vi "Close Write Reference.vi"(8 "error in":errorcluster, 11 "TDMS in":refnum<class "TDMS.lvclass">) -> (0 "error out":errorcluster, 3 "TDMS out":refnum<class "TDMS.lvclass">)   [LabVIEW 2019, in "TDMS.lvlib" / "TDMS.lvclass"]
uses:
  TDMS.lvclass
  C:/Users/Public/Documents/Development/builds/Tools/Report.lvlibp/Report.lvclass
  TDMS.lvclass/TDMS.ctl
  Accessors/Read TDMS Ref.vi
  builds/Tools/Report.lvlibp/Accessors/Write Root Path.vi
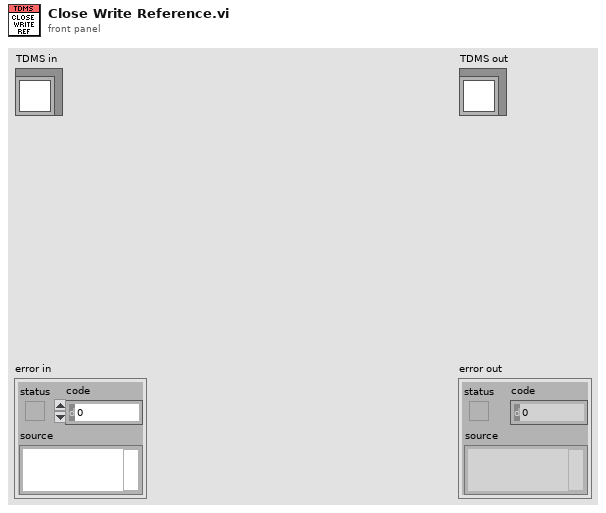
[diagram p1: front panel]
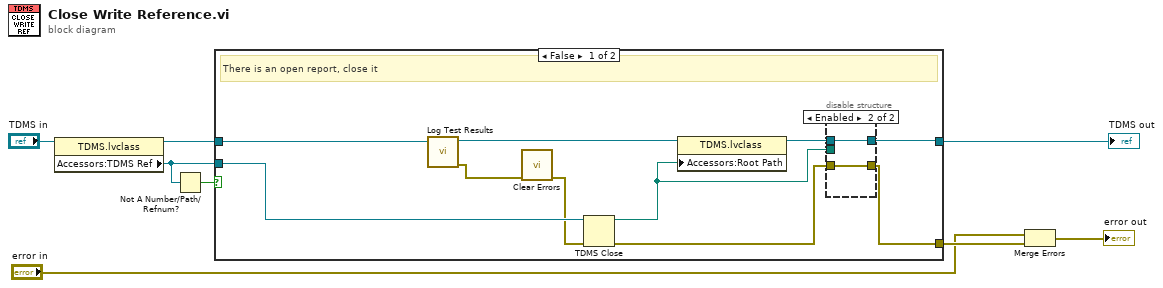
[diagram p0: block diagram]
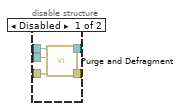
[diagram p2: hidden frame]
diagram:
  n1 = property class="TDMS.lvclass"(reference="TDMS in") -> (reference out=w5:refnum<class "TDMS.lvclass">, "Accessors:TDMS Ref"=w4:refnum<k34>)  [unwired: 1 in, 1 out]
  n2 = Not A Number/Path/Refnum?(number/path/refnum=w4) -> (NaN/Path/Refnum?=w6:bool)
  n3 = case shown="False" w6 {
    tunnel: w5 -> [w18 w26]
    tunnel: w4 -> [w17 _]
    tunnel: [w12 w26] -> w3
    tunnel: [w10 _] -> w2
    frame False {
      # "There is an open report, close it"
      n4 = call "Log Test Results.vi"("TDMS in"=w18) -> ("error out"=w14:errorcluster, "TDMS out"=w15:refnum<class "TDMS.lvclass">)  [unwired: 9 in]
      n5 = call <vilib>:"Clear Errors.vi"("error in (no error)"=w14) -> ("error out"=w16:errorcluster)  [unwired: 5 in, 1 out]
      n6 = TDMS Close(8:w16, 11:w17) -> (0:w11:errorcluster, 3:w9:path)
      n7 = property class="TDMS.lvclass"(reference=w15, "Accessors:Root Path"=w9) -> (reference out=w13:refnum<class "TDMS.lvclass">)  [unwired: 1 in, 1 out]
      n8 = disable-structure shown="Enabled" {
        disable-tunnel: w13 -> [w23 w25]
        disable-tunnel: [w22 w25] -> w12
        disable-tunnel: w11 -> [w21 w24]
        disable-tunnel: [w20 w24] -> w10
        disable-tunnel: w9 -> [w19 _]
        frame Disabled {
          n9 = call "Purge and Defragment.vi"("error in"=w21, "Path"=w19, "TDMS in"=w23) -> ("error out"=w20:errorcluster, "TDMS out"=w22:refnum<class "TDMS.lvclass">)  [unwired: 7 in]
        }
        frame Enabled {
        }
      }
    }
    frame True {
      # "There is no open report, no need to close an invalid reference"
    }
  }
  "TDMS out" <- w3
  n10 = Merge Errors("error in", w2) -> (→"error out":errorcluster)
